vi "Handle Tree Shortcut Activation Event.vi"(6 "Coords":T1, 8 "error in":errorcluster, 9 "tree refnum":refnum<vi>, 10 "menu reference":refnum<k9>, 11 "state in":T2) -> (0 "error out":errorcluster, 1 "discard?":bool, 3 "state out":T2)   [LabVIEW 2010, in "NI_SE_Config Front Panel Layout.lvlib"]
uses:
  NI_SE_Config Front Panel Layout.lvlib
  State.ctl
  VI Info.ctl
  VI Panel Layout/VI Panel Layout.lvclass
  <vilib>/Utility/miscctls.llb/LVPoint32TypeDef.ctl
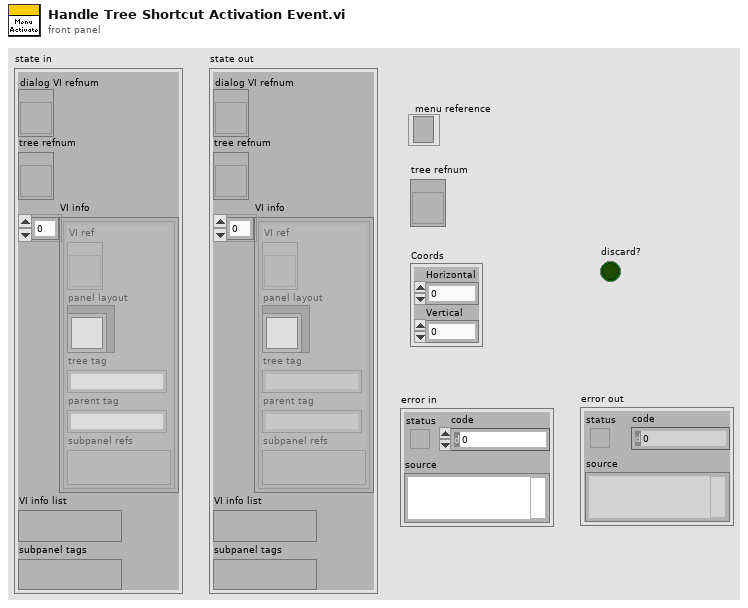
[diagram p1: front panel]
types:
  T1 = typedef "LVPoint32TypeDef.ctl" = cluster{"Horizontal":i32, "Vertical":i32}
  T2 = typedef "NI_SE_Config Front Panel Layout.lvlib/State.ctl" = cluster{"dialog VI refnum":refnum<vi>, "tree refnum":refnum<vi>, "VI info":T3[], "VI info list":variant, "subpanel tags":variant}
  T3 = typedef "NI_SE_Config Front Panel Layout.lvlib/VI Info.ctl" = cluster{"VI ref":refnum<vi>, "panel layout":refnum<class "VI Panel Layout.lvclass">, "tree tag":string, "parent tag":string, "subpanel refs":variant}
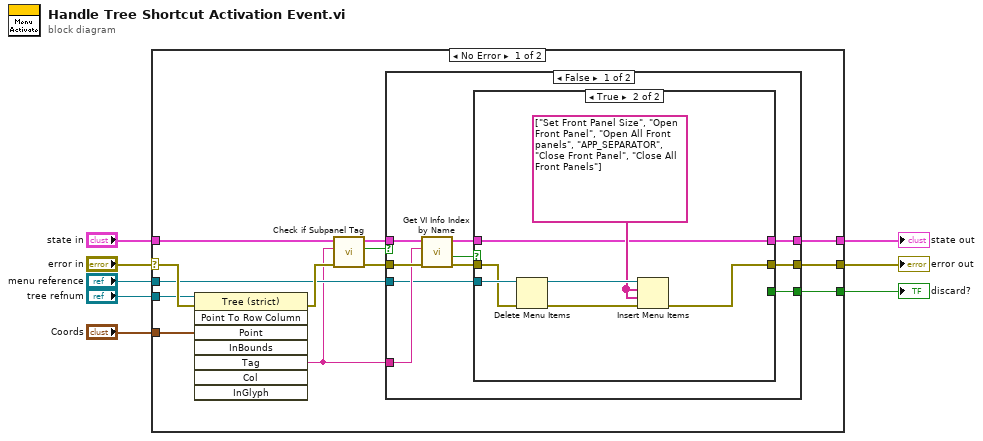
[diagram p0: block diagram]
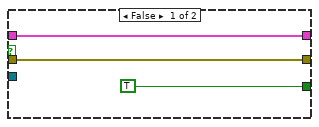
[diagram p2: hidden frame]
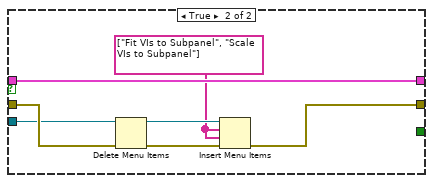
[diagram p3: hidden frame]
diagram:
  n1 = case shown="No Error" "error in" {
    selector: "error in" -> [w17 w49]
    tunnel: "state in" -> [w18 w50]
    tunnel: [w12 w50] -> w6
    tunnel: [w11 w49] -> w5
    tunnel: "menu reference" -> [w15 _]
    tunnel: "tree refnum" -> [w14 _]
    tunnel: "Coords" -> [w13 _]
    tunnel: [w10 _] -> w2
    frame No Error {
      n2 = invoke class="Tree (strict)" method="Point To Row Column"(reference=w14, error in=w17, "Point"=w13) -> (error out=w16:errorcluster, "Tag"=w9:string)  [unwired: 5 in, 6 out]
      n3 = call "Check if Subpanel Tag.vi"("error in"=w16, "subpanel tag"=w9, "state in"=w18) -> ("error out"=w19:errorcluster, "found?"=w21:bool, "state out"=w20:T2)  [unwired: 4 in, 2 out]
      n4 = case shown="False" w21 {
        tunnel: w20 -> [w30 w48]
        tunnel: w19 -> [w29 w45]
        tunnel: [w25 w48] -> w12
        tunnel: [w23 w44] -> w11
        tunnel: [w31 _] -> w10
        tunnel: w15 -> [w22 w42]
        tunnel: w9 -> [w28 _]
        frame False {
          n5 = call "Get VI Info Index by Name.vi"("error in"=w29, "VI name"=w28, "state in"=w30) -> ("error out"=w24:errorcluster, "found?"=w27:bool, "state out"=w26:T2)  [unwired: 5 in, 1 out]
          n6 = case shown="True" w27 {
            tunnel: [TRUE _] -> w31
            tunnel: w26 -> [w33 w37]
            tunnel: [w33 w37] -> w25
            tunnel: w24 -> [w32 w36]
            tunnel: [w32 w35] -> w23
            tunnel: w22 -> [_ w38]
            frame False {
            }
            frame True {
              w39 = string[] ["Set Front Panel Size", "Open Front Panel", "Open All Front panels", "APP_SEPARATOR", "Close Front Panel", "Close All Front Panels"]
              n7 = Delete Menu Items(6:w36, 9:w38) -> (0:w40:errorcluster, 3:w41:refnum<k9>)  [unwired: 2 in]
              n8 = Insert Menu Items(6:w40, 7:w39, 8:w39, 9:w41) -> (0:w35:errorcluster)  [unwired: 2 in, 2 out]
            }
          }
        }
        frame True {
          w43 = string[] ["Fit VIs to Subpanel", "Scale VIs to Subpanel"]
          n9 = Delete Menu Items(6:w45, 9:w42) -> (0:w46:errorcluster, 3:w47:refnum<k9>)  [unwired: 2 in]
          n10 = Insert Menu Items(6:w46, 7:w43, 8:w43, 9:w47) -> (0:w44:errorcluster)  [unwired: 2 in, 2 out]
        }
      }
    }
    frame Error {
    }
  }
  "state out" <- w6
  "error out" <- w5
  "discard?" <- w2
